vi "PhotonPoseEstimator_AddHeadingData_Rotation3d.vi"(9 "Heading":T1={"Q_quaternion"={"R"=1.0, "V"=[0.0, 0.0, 0.0]}}, 11 "TimeStamp":dbl=-1.0) -> ()   [LabVIEW 2019, in "PhotonVisionLib.lvlib"]
doc: "Add heading data\n\nInputs: \n -- TimeStamp -- double -- System elapsed time from FPGA\n -- Heading -- Rotation3d -- Heading value\n\nOutputs:\n - none -"
uses:
  PhotonVisionLib.lvlib
  <vilib>/Rock Robotics/WPI/ThirdParty/JAS_Junk/TrajLib/TypeDef/ROTATION3D.ctl
  <vilib>/Rock Robotics/WPI/ThirdParty/JAS_Junk/TrajLib/TypeDef/QUATERNION.ctl
  <vilib>/Rock Robotics/WPI/ThirdParty/JAS_Junk/TrajLib/VI/TimeInterpRotation2d_CleanUp.vi
  <vilib>/Rock Robotics/WPI/ThirdParty/JAS_Junk/TrajLib/Rotation2d_CreateAngle.vi
  <vilib>/Rock Robotics/WPI/ThirdParty/JAS_Junk/TrajLib/VI/Rotation3d_GetXYZ.vi
  <vilib>/Rock Robotics/WPI/ThirdParty/JAS_Junk/TrajLib/VI/Quaternion_Get_All.vi
  <vilib>/Rock Robotics/WPI/ThirdParty/JAS_Junk/TrajLib/VI/Rotation3d_GetQuaterion.vi
  PhotonVision_Globals.vi
  <vilib>/gmath/interp.llb/Search Ordered Table.vi
  <vilib>/Rock Robotics/WPI/ThirdParty/JAS_Junk/TrajLib/Trajectory_Library.lvlib
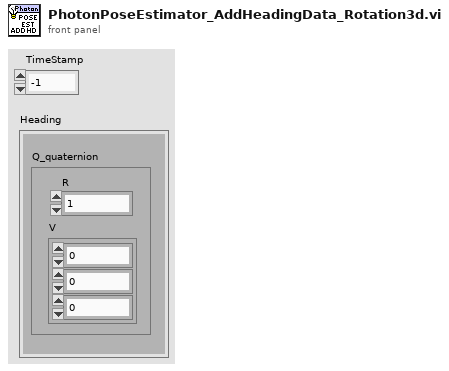
[diagram p1: front panel]
types:
  T1 = typedef "Trajectory_Library.lvlib/ROTATION3D.ctl" = cluster{"Q_quaternion":T2}
  T2 = typedef "Trajectory_Library.lvlib/QUATERNION.ctl" = cluster{"R":dbl, "V":dbl[]}
  T3 = typedef "Trajectory_Library.lvlib/TIME_INTERPOLATABLE_ROTATION2D.ctl" = cluster{"TimeStamps":dbl[], "RotationValues":T4[], "Min_TimeStamp":dbl, "Max_TimeStamp":dbl, "ItemCount":i32, "MaxBufferTime":dbl}
  T4 = typedef "Trajectory_Library.lvlib/ROTATION2D.ctl" = cluster{"VALUE":dbl, "COS":dbl, "SIN":dbl}
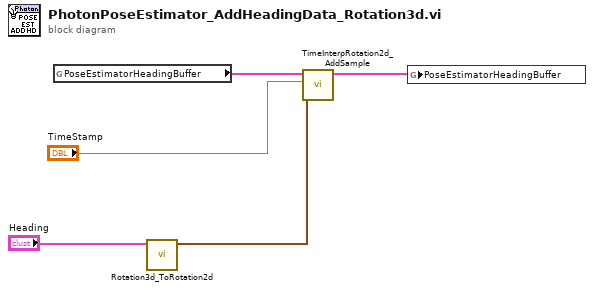
[diagram p0: block diagram]
diagram:
  n1 = global read "PhotonVision_Globals.vi" "PoseEstimatorHeadingBuffer"() -> (w5:T3)
  n2 = call <vilib>:"Rotation3d_ToRotation2d.vi"("in Rotation3d"="Heading") -> ("out Rotation2d"=w2:T4)  [unwired: 10 in]
  n3 = call <vilib>:"TimeInterpRotation2d_AddSample.vi"("RotationValue"=w2, "TimeStamp"="TimeStamp", "in TimeInterpRotation"=w5) -> ("out TimeInterpRotation"=w4:T3)  [unwired: 7 in, 1 out]
  n4 = global write "PhotonVision_Globals.vi" "PoseEstimatorHeadingBuffer"(w4) -> ()
